vi "CRYMake Name.vi"(4 "sOption 2":string, 6 "Step No.":i32, 7 "Type":enum16{"Curves", "Values", "Results", "WFM"}(ring), 8 "nData":i32[](array[numeric]), 9 "sOption":string, 10 "sAction":string, 11 "Name In":string) -> (0 "Exist?":bool, 3 "Name Out":string)   [LabVIEW 2013]
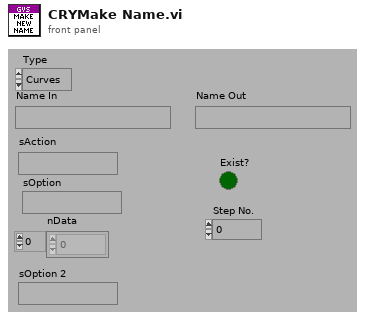
[diagram p1: front panel]
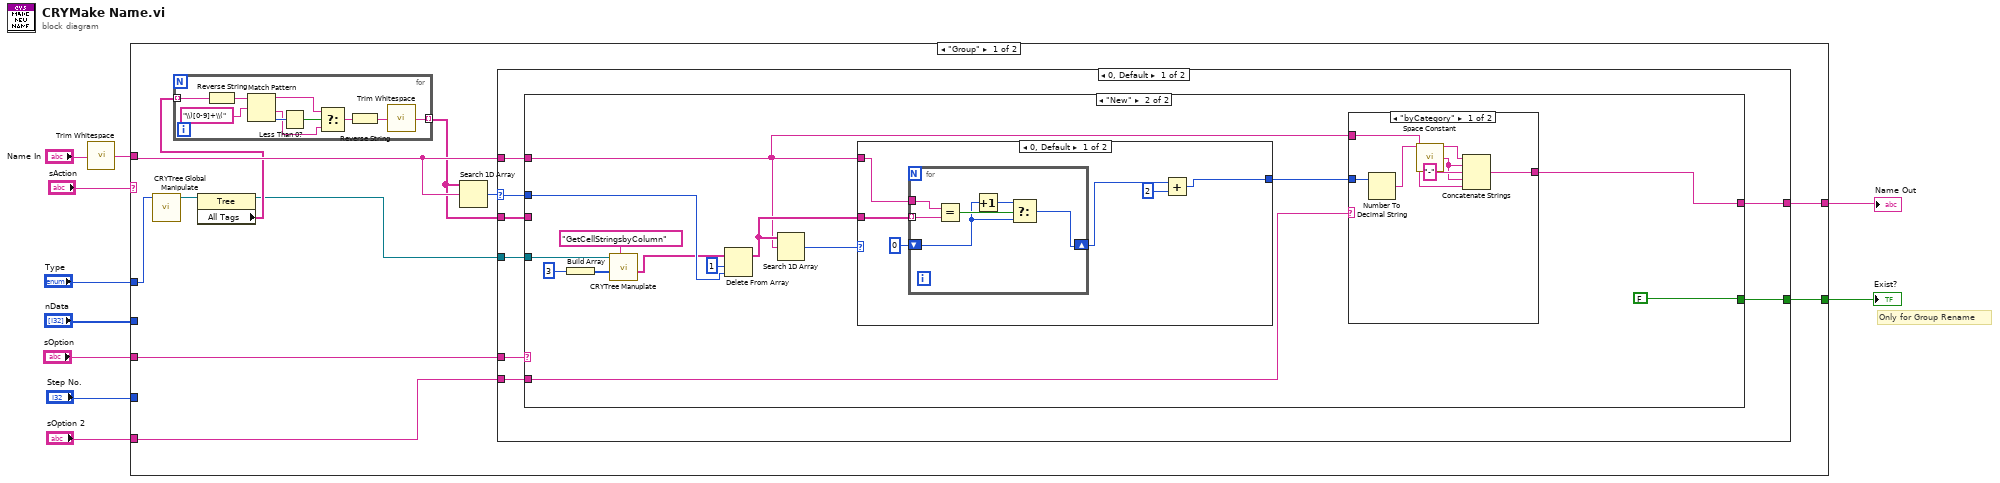
[diagram p0: block diagram]
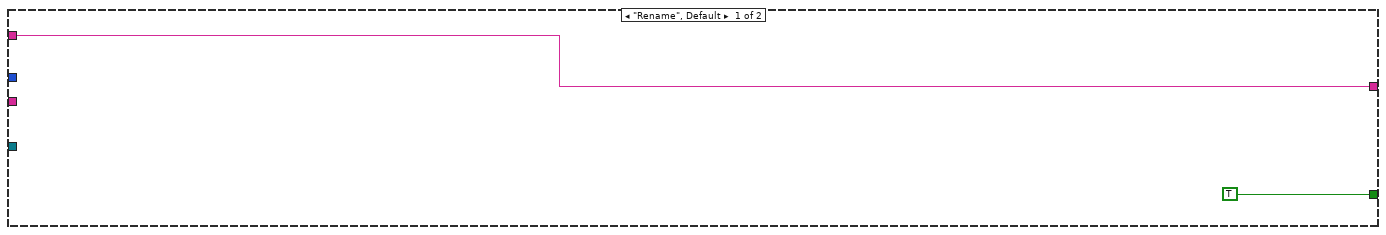
[diagram p2: hidden frame]
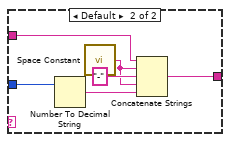
[diagram p3: hidden frame]
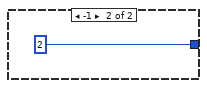
[diagram p4: hidden frame]
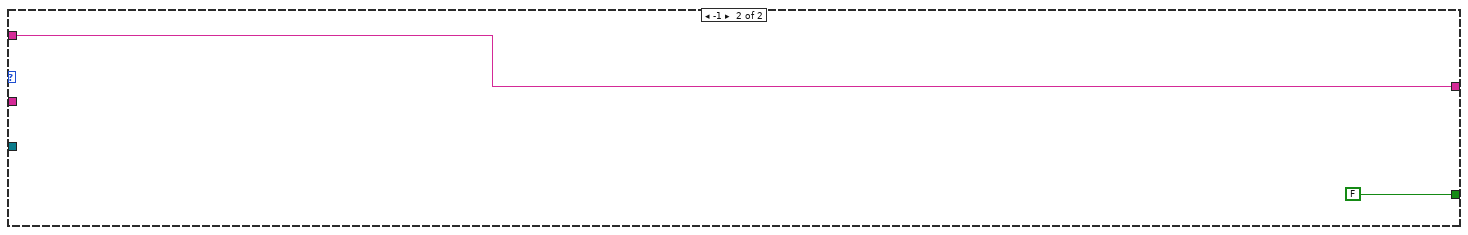
[diagram p5: hidden frame]
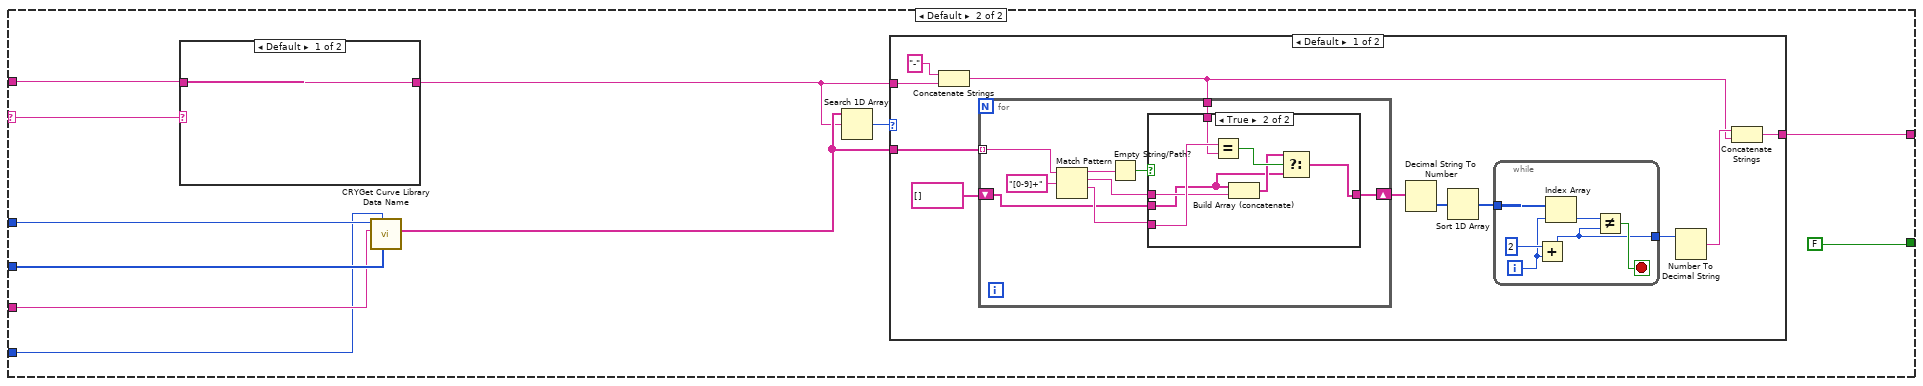
[diagram p6: hidden frame]
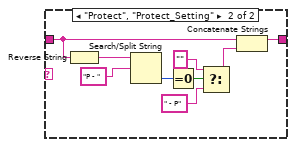
[diagram p7: hidden frame]
diagram:
  # "Only for Group Rename"
  n1 = call <vilib>:"Trim Whitespace.vi"("string"="Name In") -> ("trimmed string"=w8:string)  [unwired: 1 in]
  n2 = case shown="\"Group\"" "sAction" {
    selector: "sAction" -> [_ w84]
    tunnel: [w20 w92] -> w10
    tunnel: w8 -> [w19 w90]
    tunnel: "Type" -> [w18 w88]
    tunnel: "nData" -> [_ w87]
    tunnel: "sOption" -> [w16 w86]
    tunnel: "Step No." -> [_ w85]
    tunnel: [w13 FALSE] -> w2
    tunnel: "sOption 2" -> [w11 _]
    frame "Group" {
      n3 = call "CRYTree Global Manipulate.vi"("Type In"=w18) -> ("Tree/Curve Tree"=w17:refnum<vi>)  [unwired: 7 in, 3 out]
      n4 = property class="Tree"(reference=w17) -> (reference out=w14:refnum<vi>, "All Tags"=w15:string[])  [unwired: 1 in, 1 out]
      n5 = for {
        tunnel: [w28] -> w12 mode=indexing
        tunnel: w15 -> [w30] mode=indexing
        n6 = Reverse String(1:w30) -> (0:w25:string)
        n7 = Match Pattern(string=w25, regular expression="\\)[0-9]+\\(" ("search string/char (-)")) -> (before substring=w22:string, after substring=w24:string, offset past match=w26:i32)  [unwired: 1 in, 1 out]
        n8 = Less Than 0?(x=w26) -> (x < 0?=w27:bool)
        n9 = Select(t=w22, s=w27, f=w24) -> (s? t:f=w23:string)
        n10 = Reverse String(1:w23) -> (0:w29:string)
        n11 = call <vilib>:"Trim Whitespace.vi"("string"=w29) -> ("trimmed string"=w28:string)  [unwired: 1 in]
      }
      n12 = Search 1D Array(1D array=w12, element=w19) -> (index of element=w21:i32)  [unwired: 1 in]
      n13 = case shown="0, Default" w21 {
        selector: w21 -> [w34 _]
        tunnel: w12 -> [w39 _]
        tunnel: [w38 w82] -> w20
        tunnel: w19 -> [w37 w82]
        tunnel: w16 -> [w36 _]
        tunnel: w14 -> [w35 _]
        tunnel: [w33 FALSE] -> w13
        tunnel: w11 -> [w32 _]
        frame 0, Default {
          n14 = case shown="\"New\"" w36 {
            tunnel: w39 -> [_ _]
            tunnel: [w41 w43] -> w38
            tunnel: w37 -> [w41 w44]
            tunnel: w35 -> [_ w45]
            tunnel: w34 -> [_ w51]
            tunnel: [TRUE FALSE] -> w33
            tunnel: w32 -> [_ w42]
            frame "Rename", Default {
            }
            frame "New" {
              n15 = Build Array(3 ("nData 2")) -> (w53:i32[])
              n16 = call "CRYTree Manuplate.vi"("sAction"="GetCellStringsbyColumn", "nData"=w53, "Tree in"=w45) -> ("sData Out"=w50:string[])  [unwired: 5 in, 3 out]
              n17 = Delete From Array(array=w50, length=1, index=w51) -> (array with subset deleted=w48:string[])  [unwired: 1 out]
              n18 = Search 1D Array(1D array=w48, element=w44) -> (index of element=w49:i32)  [unwired: 1 in]
              n19 = case shown="0, Default" w49 {
                tunnel: w48 -> [w73 _]
                tunnel: w44 -> [w71 _]
                tunnel: [w70 2] -> w47
                frame 0, Default {
                  n20 = for {
                    tunnel: w73 -> [w78] mode=indexing
                    tunnel: w71 -> [w79]
                    shift-right: [w74] -> w69
                    shift-left: 0 -> [w76]
                    n21 = Equal?(x=w79, y=w78) -> (x = y?=w77:bool)
                    n22 = Increment(x=w76) -> (x+1=w75:i32)
                    n23 = Select(t=w75, s=w77, f=w76) -> (s? t:f=w74:i32)
                  }
                  n24 = Add(x=w69, y=2) -> (x+y=w70:i32)
                }
                frame -1 {
                }
              }
              n25 = case shown="\"byCategory\"" w42 {
                tunnel: w47 -> [w61 w67]
                tunnel: w44 -> [w56 w63]
                tunnel: [w58 w62] -> w43
                frame "byCategory" {
                  n26 = Number To Decimal String(number=w61) -> (decimal integer string=w57:string)  [unwired: 1 in]
                  n27 = call <vilib>:"Space Constant.vi"() -> ("String"=w59:string)
                  n28 = Concatenate Strings(w57, w59, "-" ("string"), w59, w56) -> (w58:string)
                }
                frame Default {
                  n29 = Number To Decimal String(number=w67) -> (decimal integer string=w64:string)  [unwired: 1 in]
                  n30 = call <vilib>:"Space Constant.vi"() -> ("String"=w65:string)
                  n31 = Concatenate Strings(w63, w65, "-" ("string"), w65, w64) -> (w62:string)
                }
              }
            }
          }
        }
        frame -1 {
        }
      }
    }
    frame Default {
      n32 = case shown="Default" w84 {
        tunnel: [w94 w103] -> w89
        tunnel: w90 -> [w94 w102]
        frame Default {
        }
        frame "Protect", "Protect_Setting" {
          n33 = Reverse String(1:w102) -> (0:w100:string)
          n34 = Search/Split String(string=w100, search string/char (-)="P - " ("element")) -> (offset of match=w99:i32)  [unwired: 1 in, 2 out]
          n35 = Equal To 0?(x=w99) -> (x = 0?=w98:bool)
          n36 = Select(t="" ("string"), s=w98, f=" - P" ("element")) -> (s? t:f=w95:string)
          n37 = Concatenate Strings(w102, w95) -> (w103:string)
        }
      }
      n38 = call "CRYGet Curve Library Data Name.vi"("nData"=w87, "Step No."=w85, "sAction"=w86, "Type"=w88) -> ("sNames"=w91:string[])  [unwired: 4 in, 3 out]
      n39 = Search 1D Array(1D array=w91, element=w89) -> (index of element=w93:i32)  [unwired: 1 in]
      n40 = case shown="Default" w93 {
        tunnel: w91 -> [w114 _]
        tunnel: [w108 w138] -> w92
        tunnel: w89 -> [w106 w138]
        frame Default {
          n41 = Concatenate Strings("-" ("element"), w106) -> (w104:string)
          n42 = for {
            tunnel: w114 -> [w119] mode=indexing
            shift-right: [w118] -> w113
            shift-left: string[] [] -> [w117]
            tunnel: w104 -> [w115]
            n43 = Match Pattern(string=w119, regular expression="[0-9]+") -> (before substring=w122:string, match substring=w116:string, after substring=w120:string)  [unwired: 1 in, 1 out]
            n44 = Empty String/Path?(string/path=w122) -> (empty?=w121:bool)
            n45 = case shown="True" w121 {
              tunnel: w120 -> [_ w131]
              tunnel: w116 -> [_ w130]
              tunnel: [w124 w126] -> w118
              tunnel: w117 -> [w124 w127]
              tunnel: w115 -> [_ w125]
              frame False {
              }
              frame True {
                n46 = Equal?(x=w131, y=w125) -> (x = y?=w129:bool)
                n47 = Build Array (concatenate)(w127, w130) -> (w128:string[])
                n48 = Select(t=w128, s=w129, f=w127) -> (s? t:f=w126:string[])
              }
            }
          }
          n49 = Decimal String To Number(string=w113) -> (number=w112:i32[])  [unwired: 2 in, 1 out]
          n50 = Sort 1D Array(array=w112) -> (sorted array=w111:i32[])
          n51 = while {
            tunnel: w111 -> [w135]
            tunnel: [w132] -> w110
            i -> [w134]
            stop <- w136 stop-if-true
            n52 = Add(x=2, y=w134) -> (x+y=w132:i32)
            n53 = Index Array(array=w135, index=w134) -> (element=w133:i32)
            n54 = Not Equal?(x=w133, y=w132) -> (x != y?=w136:bool)
          }
          n55 = Number To Decimal String(number=w110) -> (decimal integer string=w109:string)  [unwired: 1 in]
          n56 = Concatenate Strings(w109, w104) -> (w108:string)
        }
        frame -1 {
        }
      }
    }
  }
  "Name Out" <- w10
  "Exist?" <- w2
